vi "MSScript_SubVI_ArrayVarSetValue.vi"(10 "ArrayValue in":ext[](array[numeric]), 11 "VarString in":string) -> (2 "Value Error?":bool, 3 "isVar?":bool)   [LabVIEW 2018, in "MSScript.lvclass"]
uses:
  MSScript.lvclass
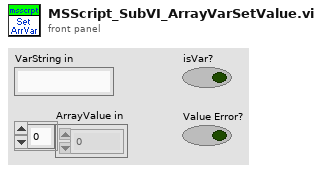
[diagram p1: front panel]
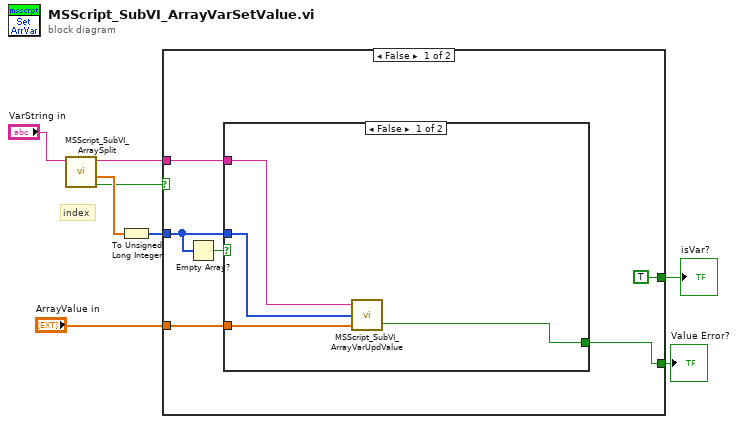
[diagram p0: block diagram]
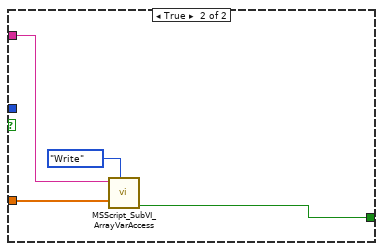
[diagram p2: hidden frame]
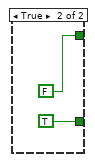
[diagram p3: hidden frame]
diagram:
  # "index"
  n1 = call "MSScript_SubVI_ArraySplit.vi"("VarString in"="VarString in") -> ("Value Error?"=w2:bool, "ArrayVariable out"=w7:ext[], "@name"=w6:string)  [unwired: 7 in, 1 out]
  n2 = To Unsigned Long Integer(number=w7) -> (unsigned 32bit integer=w8:u32[])
  n3 = case shown="False" w2 {
    tunnel: "ArrayValue in" -> [w13 _]
    tunnel: [TRUE FALSE] -> w4
    tunnel: [w10 TRUE] -> w5
    tunnel: w8 -> [w12 _]
    tunnel: w6 -> [w11 _]
    frame False {
      n4 = Empty Array?(array=w12) -> (empty?=w14:bool)
      n5 = case shown="False" w14 {
        tunnel: w13 -> [w16 w21]
        tunnel: w12 -> [w18 _]
        tunnel: w11 -> [w17 w19]
        tunnel: [w15 w20] -> w10
        frame False {
          n6 = call "MSScript_SubVI_ArrayVarUpdValue.vi"("new variable"=w16, "index arr"=w18, "@name"=w17) -> ("error"=w15:bool)  [unwired: 1 in]
        }
        frame True {
          n7 = call "MSScript_SubVI_ArrayVarAccess.vi"("Function (Read)"=enum16{"Init", "Write", "Read"}."Write", "ArrayVariable in"=w21, "VarName"=w19) -> ("Value Error?"=w20:bool)  [unwired: 4 in, 2 out]
        }
      }
    }
    frame True {
    }
  }
  "Value Error?" <- w5
  "isVar?" <- w4
